vi "Exec State to Append.vi"(3 "Execution:State":T1(ring)) -> (1 "append?":bool)   [LabVIEW 2019, in "Transport.lvclass"]
uses:
  Transport.lvclass
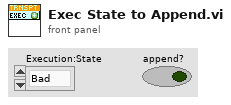
[diagram p1: front panel]
types:
  T1 = enum32{"Bad", "Idle", "Run top level", "Running"}
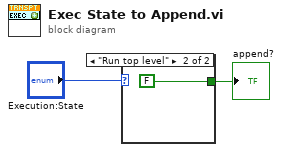
[diagram p0: block diagram]
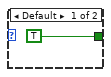
[diagram p2: hidden frame]
diagram:
  n1 = case shown="\"Run top level\"" "Execution:State" {
    tunnel: [TRUE ("append?") FALSE ("append?")] -> w1
    frame Default {
    }
    frame "Run top level" {
    }
  }
  "append?" <- w1
